vi "Get Pythonic Function Call.vi"(8 "Error In":errorcluster, 10 "Function Name":string, 11 "Arg Dict":variant) -> (0 "Error Out":errorcluster, 2 "Function Call":string)   [LabVIEW 2016, in "OPI.lvclass"]
uses:
  OPI.lvclass
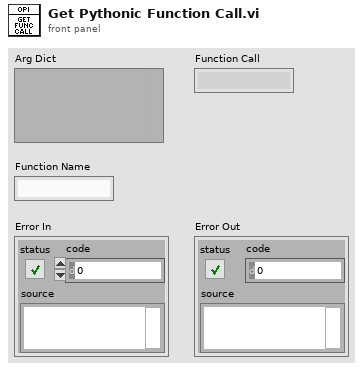
[diagram p1: front panel]
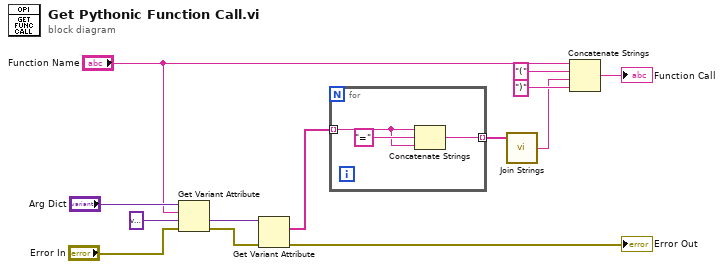
[diagram p0: block diagram]
diagram:
  n1 = Get Variant Attribute(Variant="Arg Dict", name="Function Name", default value (empty Variant)=variant ("variant"), error in="Error In") -> (value=w11:variant, error out=w13:errorcluster)  [unwired: 2 out]
  n2 = Get Variant Attribute(Variant=w11, error in=w13) -> (names=w7:string[], error out=→"Error Out":errorcluster)  [unwired: 2 in, 2 out]
  n3 = for {
    tunnel: w7 -> [w15] mode=indexing
    tunnel: [w14] -> w6 mode=indexing
    n4 = Concatenate Strings(w15, "=" ("string"), w15) -> (w14:string)
  }
  n5 = call <vilib>:"Join Strings.vi"("Strings In"=w6) -> ("String"=w3:string)  [unwired: 2 in]
  n6 = Concatenate Strings("Function Name", "(" ("string"), w3, ")" ("string")) -> (→"Function Call":string)
